vi "READBMSDYNDATA.vi"(8 "errin":errorcluster, 10 "set 400?":bool, 11 "Channel out":T1) -> (0 "errout":errorcluster, 3 "Data out":T2)   [LabVIEW 2020]
uses:
  PCAN Basic/Controls/Channel.ctl
  PCAN Basic/Controls/BaudrateEenum.ctl
  PCAN Basic/PCANBasic.lvlib
  Alex_Peak_lib/PEAK_lib_ALEX.lvlib
panel:
  out "F106 Power Distribution Status":string
  out "stop":bool
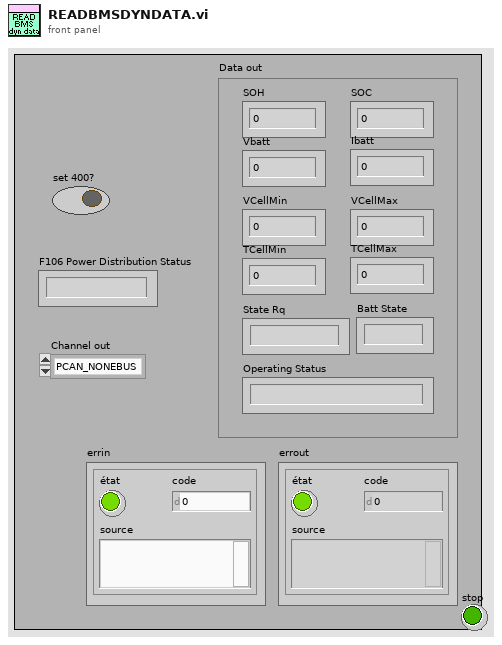
[diagram p1: front panel]
types:
  T1 = typedef "PCANBasic.lvlib/Channel.ctl" = enum16{"PCAN_NONEBUS", "not used1", "not used2", "not used3", "not used4", "not used5", "not used6", "not used7", "not used8", "not used9", "not used10", "not used11", "not used12", "not used13", "not used14", "not used15", "not used16", "not used17", "not used18", "not used19", "not used20", "not used21", "not used22", "not used23", "not used24", "not used25", "not used26", "not used27", "not used28", "not used29", "not used30", "not used31", "not used32", "PCAN_ISABUS1", "PCAN_ISABUS2", "PCAN_ISABUS3", "PCAN_ISABUS4", "PCAN_ISABUS5", "PCAN_ISABUS6", "PCAN_ISABUS7", "PCAN_ISABUS8", "not used41", "not used42", "not used43", "not used44", "not used45", "not used46", "not used47", "not used48", "PCAN_DNGBUS1", "not used50", "not used51", "not used52", "not used53", "not used54", "not used55", "not used56", "not used57", "not used58", "not used59", "not used60", "not used61", "not used62", "not used63", "not used64", "PCAN_PCIBUS1", "PCAN_PCIBUS2", "PCAN_PCIBUS3", "PCAN_PCIBUS4", "PCAN_PCIBUS5", "PCAN_PCIBUS6", "PCAN_PCIBUS7", "PCAN_PCIBUS8", "not used73", "not used74", "not used75", "not used76", "not used77", "not used78", "not used79", "not used80", "PCAN_USBBUS1", "PCAN_USBBUS2", "PCAN_USBBUS3", "PCAN_USBBUS4", "PCAN_USBBUS5", "PCAN_USBBUS6", "PCAN_USBBUS7", "PCAN_USBBUS8", "Not used89", "Not used90", "Not used91", "Not used92", "Not used93", "Not used94", "Not used95", "Not used96", "PCAN_PCCBUS1", "PCAN_PCCBUS2"}
  T2 = cluster{"SOH":dbl, "SOC":dbl, "Vbatt":u32, "Ibatt":dbl, "VCellMax":u32, "VCellMin":u32, "TCellMin":i32, "TCellMax":i32, "State Rq":string, "Batt State":string, "Operating Status":string}
  T3 = typedef "PCANBasic.lvlib/BaudrateEenum.ctl" = enum16{"CAN_Baud_1M", "CAN_Baud_800K", "CAN_BAUD_500K", "CAN_BAUD_250K", "CAN_BAUD_125K", "CAN_BAUD_100K", "CAN_BAUD_95K", "CAN_BAUD_83K", "CAN_BAUD_50K", "CAN_BAUD_47K", "CAN_BAUD_33K", "CAN_BAUD_20K", "CAN_BAUD_10K", "CAN_BAUD_5K", "User Baudrate"}
  T4 = cluster{"F400 Battery Charge Type":string, "F400 Battery State Request":string, "F400 Ext Insulation Test Control":string, "F400 Int Insulation Test Control":string, "F400 Vehicle Speed":i32, "F400 Ambiant Temperature":i32, "F400 Charger Available Power":i32, "F400 Count":i32, "F106 Keep Active request":string, "F106 Battery State":string, "F106 Operating Status":string, "F106 Battery SOC":dbl, "F106 Battery SOH":dbl, "F106 Ext Insulation Test Status":string, "F106 Int Insulation Test Status":string, "F106 Power Distribution Status":string, "F106 Power Switch Off Delay":i32, "F106 Power Switch Off Request":string, "F106 Count":i32, "F101 Battery Voltage":u32, "F101 Battery Current":dbl, "F101 Max Charge Current":u32, "F101 Max Discharge Current":u32, "F101 Max Discharge Current Temp Limit":string, "F101 Max Discharge Current SOC Limit":string, "F101 Max Charge Current Temp Limit":string, "F101 Max Charge Current SOC Limit":string, "F101 Deliverable Energy":dbl, "F101 Count":u32, "F102 Cell Average Voltage":u32, "F102 Cell Min Voltage":u32, "F102 Cell Max Voltage":u32, "F102 Cell Average Temp":i32, "F102 Cell Min Temp":i32, "F102 Count":u32, "F103 SumOfInternalResistanceT":i32, "F100 Charge Voltage Setpoint":i32, "F100 Charge Current Setpoint":dbl, "F100 Equilization Status":bool, "F100 Charge Competed":bool, "F100 Count":i32, "F107 Outlet Water Temp Request":i32, "F107 Outlet Water Temp Status":i32, "F107 Flow Rate Request":i32, "F107 Inlet Water Temp":i32, "F107 Ambiant Temperature 2":i32, "F105 Max Power Charge Continuous":i32, "F105 Max Power Charge Long Prediction":i32, "F105 Max Power Charge Short Prediction":i32, "F105 Max Current Charge Continuous":i32, "F105 Max Current Charge Short Prediction":i32, "F105 Count ":i32, "F104 Max Power Discharge Continuous":i32, "F104 Max Power Discharge Long Prediction":i32, "F104 Max Power Discharge Short Prediction":i32, "F104 Max Current Discharge Continuous":i32, "F104 Max Current Discharge Short Prediction":i32, "F104 Count ":i32, "F103 Count":i32, "F103 Cell Max Temp":i32, "F103 Max Current Discharge Long Prediction":i32, "F103 Max Current Charge Long Prediction":i32, "F107 Count":i32}
  T5 = cluster{"ID":u32, "MSGTYPE":u8, "LEN":u8, "DATA[0]":u8, "DATA[1]":u8, "DATA[2]":u8, "DATA[3]":u8, "DATA[4]":u8, "DATA[5]":u8, "DATA[6]":u8, "DATA[7]":u8}
  T6 = cluster{"F400 Battery Charge Type":string, "F400 Battery State Request":string, "F400 Ext Insulation Test Control":string, "F400 Int Insulation Test Control":string, "F400 Vehicle Speed":i32, "F400 Ambiant Temperature":i32, "F400 Charger Available Power":i32, "F400 Count":i32, "F106 Keep Active request":string, "F106 Battery State":string, "F106 Operating Status":string, "F106 Battery SOC":dbl, "F106 Battery SOH":dbl, "F106 Ext Insulation Test Status":string, "F106 Int Insulation Test Status":string, "F106 Power Distribution Status":string, "F106 Power Switch Off Delay":i32, "F106 Power Switch Off Request":string, "F106 Count":i32, "F101 Battery Voltage":u32, "F101 Battery Current":dbl, "F101 Max Charge Current":u32, "F101 Max Discharge Current":u32, "F101 Max Discharge Current Temp Limit":string, "F101 Max Discharge Current SOC Limit":string, "F101 Max Charge Current Temp Limit":string, "F101 Max Charge Current SOC Limit":string, "F101 Deliverable Energy":dbl, "F101 Count":u32, "F102 Cell Average Voltage":u32, "F102 Cell Min Voltage":u32, "F102 Cell Max Voltage":u32, "F102 Cell Average Temp":i32, "F102 Cell Min Temp":i32, "F102 Count":u32, "F103 SumOfInternalResistanceT":i32, "F100 Charge Voltage Setpoint":i32, "F100 Charge Current Setpoint":i32, "F100 Equilization Status":bool, "F100 Charge Competed":bool, "F100 Count":i32, "F107 Outlet Water Temp Request":i32, "F107 Outlet Water Temp Status":i32, "F107 Flow Rate Request":i32, "F107 Inlet Water Temp":i32, "F107 Ambiant Temperature 2":i32, "F105 Max Power Charge Continuous":i32, "F105 Max Power Charge Long Prediction":i32, "F105 Max Power Charge Short Prediction":i32, "F105 Max Current Charge Continuous":i32, "F105 Max Current Charge Short Prediction":i32, "F105 Count ":i32, "F104 Max Power Discharge Continuous":i32, "F104 Max Power Discharge Long Prediction":i32, "F104 Max Power Discharge Short Prediction":i32, "F104 Max Current Discharge Continuous":i32, "F104 Max Current Discharge Short Prediction":i32, "F104 Count ":i32, "F103 Count":i32, "F103 Cell Max Temp":i32, "F103 Max Current Discharge Long Prediction":i32, "F103 Max Current Charge Long Prediction":i32, "F107 Count":i32}
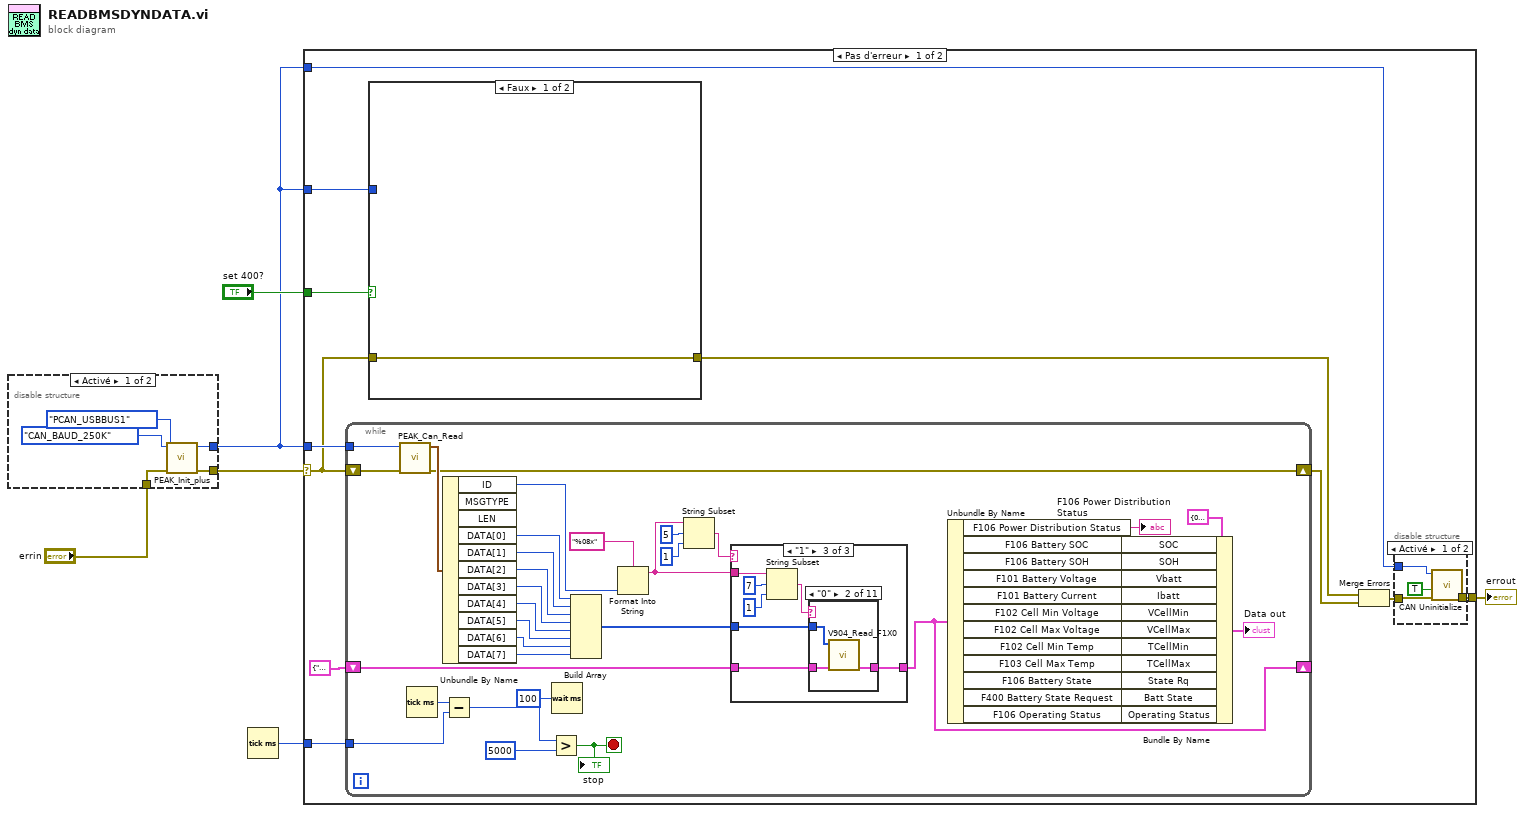
[diagram p0: block diagram]
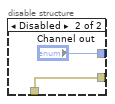
[diagram p2: hidden frame]
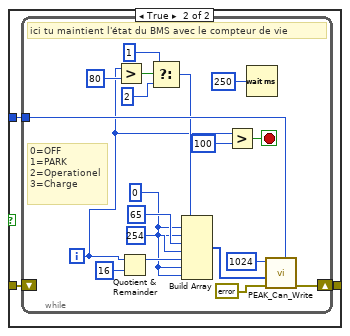
[diagram p4: hidden frame]
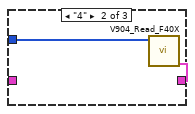
[diagram p6: hidden frame]
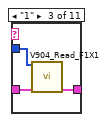
[diagram p8: hidden frame]
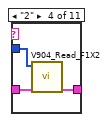
[diagram p9: hidden frame]
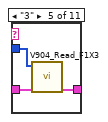
[diagram p10: hidden frame]
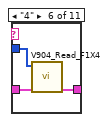
[diagram p11: hidden frame]
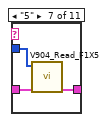
[diagram p12: hidden frame]
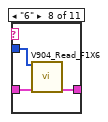
[diagram p13: hidden frame]
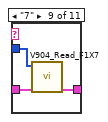
[diagram p14: hidden frame]
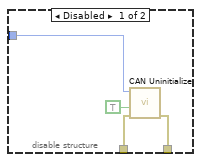
[diagram p18: hidden frame]
diagram:
  n1 = disable-structure shown="Activé" {
    disable-tunnel: [w10 w12] -> w6
    disable-tunnel: "errin" -> [w9 w12]
    disable-tunnel: [w8 "Channel out"] -> w1
    frame Enabled {
      n2 = call "PEAK_Init_plus.vi"("errin"=w9, "Channel"=Channel."PCAN_USBBUS1", "BTR0BTR1"=BaudrateEenum."CAN_BAUD_250K") -> ("errout"=w10:errorcluster, "Channel out"=w8:T1)  [unwired: 7 in]
    }
    frame Disabled {
    }
  }
  n3 = Tick Count (ms)() -> (millisecond timer value=w3:u32)
  n4 = case shown="Pas d'erreur" w6 {
    selector: w6 -> [w20 w133]
    tunnel: w1 -> [w24 w131]
    tunnel: [w21 w132] -> w5
    tunnel: w3 -> [w22 _]
    tunnel: "set 400?" -> [w19 _]
    tunnel: w1 -> [w15 _]
    tunnel: w1 -> [w14 _]
    frame No Error {
      n5 = while {
        tunnel: w24 -> [w55]
        shift-right: [w61] -> _
        shift-left: T4 {"F400 Battery Charge Type"="", "F400 Battery State Request"="", "F400 Ext Insulation Test Control"="", "F400 Int Insulation Test Control"="", "F400 Vehicle Speed"=0, "F400 Ambiant Temperature"=0, "F400 Charger Available Power"=0, "F400 Count"=0, "F106 Keep Active request"="", "F106 Battery State"="", "F106 Operating Status"="", "F106 Battery SOC"=0.0, "F106 Battery SOH"=0.0, "F106 Ext Insulation Test Status"="", "F106 Int Insulation Test Status"="", "F106 Power Distribution Status"="", "F106 Power Switch Off Delay"=0, "F106 Power Switch Off Request"="", "F106 Count"=0, "F101 Battery Voltage"=0, "F101 Battery Current"=0.0, "F101 Max Charge Current"=0, "F101 Max Discharge Current"=0, "F101 Max Discharge Current Temp Limit"="", "F101 Max Discharge Current SOC Limit"="", "F101 Max Charge Current Temp Limit"="", "F101 Max Charge Current SOC Limit"="", "F101 Deliverable Energy"=0.0, "F101 Count"=0, "F102 Cell Average Voltage"=0, "F102 Cell Min Voltage"=0, "F102 Cell Max Voltage"=0, "F102 Cell Average Temp"=0, "F102 Cell Min Temp"=0, "F102 Count"=0, "F103 SumOfInternalResistanceT"=0, "F100 Charge Voltage Setpoint"=0, "F100 Charge Current Setpoint"=0.0, "F100 Equilization Status"=FALSE, "F100 Charge Competed"=FALSE, "F100 Count"=0, "F107 Outlet Water Temp Request"=0, "F107 Outlet Water Temp Status"=0, "F107 Flow Rate Request"=0, "F107 Inlet Water Temp"=0, "F107 Ambiant Temperature 2"=0, "F105 Max Power Charge Continuous"=0, "F105 Max Power Charge Long Prediction"=0, "F105 Max Power Charge Short Prediction"=0, "F105 Max Current Charge Continuous"=0, "F105 Max Current Charge Short Prediction"=0, "F105 Count "=0, "F104 Max Power Discharge Continuous"=0, "F104 Max Power Discharge Long Prediction"=0, "F104 Max Power Discharge Short Prediction"=0, "F104 Max Current Discharge Continuous"=0, "F104 Max Current Discharge Short Prediction"=0, "F104 Count "=0, "F103 Count"=0, "F103 Cell Max Temp"=0, "F103 Max Current Discharge Long Prediction"=0, "F103 Max Current Charge Long Prediction"=0, "F107 Count"=0} ("cluster de sortie") -> [w77]
        shift-right: [w75] -> w16
        shift-left: w20 -> [w54]
        tunnel: w22 -> [w59]
        stop <- w56 stop-if-true
        n6 = call "PEAK_Can_Read.vi"("errin"=w54, "Channel out"=w55) -> ("errout"=w75:errorcluster, "MessageBuffer out"=w93:T5)  [unwired: 7 in, 1 out]
        n7 = Tick Count (ms)() -> (millisecond timer value=w60:u32)
        n8 = Unbundle By Name(w93) -> ("ID"=w87:u32, "DATA[0]"=w86:u8, "DATA[1]"=w85:u8, "DATA[2]"=w84:u8, "DATA[3]"=w83:u8, "DATA[4]"=w82:u8, "DATA[5]"=w81:u8, "DATA[6]"=w80:u8, "DATA[7]"=w79:u8)  [unwired: 2 out]
        n9 = Subtract(x=w60, y=w59) -> (x-y=w58:u32)
        n10 = Greater?(x=w58, y=u32 5000) -> (0:w56:bool)
        "stop" <- w56
        n11 = Wait (ms)(milliseconds to wait=u32 100 ("attente (ms)")) -> ()  [unwired: 1 out]
        n12 = Build Array(w86, w85, w84, w83, w82, w81, w80, w79) -> (w78:u8[])
        n13 = Format Into String(format string="%08x", w87) -> (resulting string=w91:string)  [unwired: 2 in, 1 out]
        n14 = String Subset(string=w91, offset (0)=5, length (rest)=1 ("longueur (reste)")) -> (substring=w90:string)
        n15 = case shown="\"1\"" w90 {
          tunnel: w77 -> [w94 _ w98]
          tunnel: w78 -> [_ w96 w103]
          tunnel: [w94 w95 w97] -> w61
          tunnel: w91 -> [_ _ w99]
          frame "Faux", Default {
          }
          frame "4" {
            n16 = call "V904_Read_F40X.vi"("Data"=w96) -> ("cluster de sortie"=w95:T4)  [unwired: 10 in]
          }
          frame "1" {
            n17 = String Subset(string=w99, offset (0)=7, length (rest)=1 ("longueur (reste)")) -> (substring=w100:string)
            n18 = case shown="\"0\"" w100 {
              tunnel: w103 -> [_ w107 w109 w113 w116 w119 w122 w125 w128 _ _]
              tunnel: w98 -> [w104 w106 w110 w112 w115 w118 w121 w124 w127 w129 w130]
              tunnel: [w104 w105 w108 w111 w114 w117 w120 w123 w126 w129 w130] -> w97
              frame "Faux", Default {
              }
              frame "0" {
                n19 = call "V904_Read_F1X0.vi"("cluster input"=w106, "Data"=w107) -> ("cluster de sortie"=w105:T6)  [unwired: 9 in]
              }
              frame "1" {
                n20 = call "V904_Read_F1X1.vi"("Data"=w109, "cluster input"=w110) -> ("cluster de sortie"=w108:T4)  [unwired: 13 in]
              }
              frame "2" {
                n21 = call "V904_Read_F1X2.vi"("cluster input"=w112, "Data"=w113) -> ("cluster de sortie"=w111:T4)  [unwired: 9 in]
              }
              frame "3" {
                n22 = call "V904_Read_F1X3.vi"("cluster input"=w115, "Data"=w116) -> ("cluster de sortie"=w114:T4)  [unwired: 9 in]
              }
              frame "4" {
                n23 = call "V904_Read_F1X4.vi"("cluster input"=w118, "Data"=w119) -> ("cluster de sortie"=w117:T4)  [unwired: 9 in]
              }
              frame "5" {
                n24 = call "V904_Read_F1X5.vi"("cluster input"=w121, "Data"=w122) -> ("cluster de sortie"=w120:T4)  [unwired: 9 in]
              }
              frame "6" {
                n25 = call "V904_Read_F1X6.vi"("Data"=w125, "cluster input"=w124) -> ("cluster de sortie"=w123:T4)  [unwired: 13 in]
              }
              frame "7" {
                n26 = call "V904_Read_F1X7.vi"("cluster input"=w127, "Data"=w128) -> ("cluster de sortie"=w126:T4)  [unwired: 9 in]
              }
              frame "8" {
              }
              frame "9" {
              }
            }
          }
        }
        n27 = Unbundle By Name(w61) -> ("F106 Power Distribution Status"=→"F106 Power Distribution Status":string, "F106 Battery SOC"=w73:dbl, "F106 Battery SOH"=w72:dbl, "F101 Battery Voltage"=w71:u32, "F101 Battery Current"=w70:dbl, "F102 Cell Min Voltage"=w69:u32, "F102 Cell Max Voltage"=w68:u32, "F102 Cell Min Temp"=w67:i32, "F103 Cell Max Temp"=w66:i32, "F106 Battery State"=w65:string, "F400 Battery State Request"=w64:string, "F106 Operating Status"=w63:string)
        n28 = Bundle By Name(cluster=T2 {"SOH"=0.0, "SOC"=0.0, "Vbatt"=0, "Ibatt"=0.0, "VCellMax"=0, "VCellMin"=0, "TCellMin"=0, "TCellMax"=0, "State Rq"="", "Batt State"="", "Operating Status"=""} ("Data out"), "SOC"=w73, "SOH"=w72, "Vbatt"=w71, "Ibatt"=w70, "VCellMin"=w69, "VCellMax"=w68, "TCellMin"=w67, "TCellMax"=w66, "State Rq"=w65, "Batt State"=w64, "Operating Status"=w63) -> (→"Data out":T2)
      }
      n29 = case shown="Faux" w19 {
        tunnel: w20 -> [w30 w33]
        tunnel: [w30 w32] -> w17
        tunnel: w15 -> [_ w31]
        frame False {
        }
        frame True {
          n30 = while {
            shift-right: [w52] -> w32
            shift-left: w33 -> [_]
            tunnel: w31 -> [w42]
            i -> [w36]
            stop <- w34 stop-if-true
            w43 = u8 0
            # "0=OFF\n1=PARK\n2=Operationel\n3=Charge"
            # "ici tu maintient l'état du BMS avec le compteur de vie"
            n31 = Greater?(x=w36, y=80) -> (0:w40:bool)
            n32 = Quotient & Remainder(x=w36, y=16) -> (x-y*floor(x/y)=w45:i32)  [unwired: 1 out]
            n33 = Select(t=1 ("cas vrai"), s=w40, f=2 ("élément")) -> (s? t:f=w37:i32)
            n34 = Build Array(w37, w43, w43, u8 65, u8 254, w45, w43, w43) -> (w46:i32[])
            n35 = Greater?(x=w36, y=100) -> (0:w34:bool)
            n36 = Wait (ms)(milliseconds to wait=u32 250 ("attente (ms)")) -> ()  [unwired: 1 out]
            n37 = call "PEAK_Can_Write.vi"("CAN Handle"=w42, "errin"=errorcluster {"status"=FALSE, "code"=0, "source"=""} ("errout"), "CAN Data"=w46, "Identifier"=u32 1024) -> ("errout"=w52:errorcluster)  [unwired: 7 in]
          }
        }
      }
      n38 = Merge Errors(w17, w16) -> (w18:errorcluster)
      n39 = disable-structure shown="Activé" {
        disable-tunnel: [w27 w29] -> w21
        disable-tunnel: w18 -> [w26 w29]
        disable-tunnel: w14 -> [w25 _]
        frame Enabled {
          n40 = call "CAN Uninitialize.vi"("error in (no error)"=w26, "Ignore input error"=TRUE, "Channel"=w25) -> ("error out"=w27:errorcluster)  [unwired: 6 in, 2 out]
        }
        frame Disabled {
        }
      }
    }
    frame Error {
      n41 = disable-structure shown="Activé" {
        disable-tunnel: w133 -> [w137 w138]
        disable-tunnel: [w136 w138] -> w132
        disable-tunnel: w131 -> [w134 _]
        frame Disabled {
          n42 = call "CAN Uninitialize.vi"("error in (no error)"=w137, "Ignore input error"=TRUE, "Channel"=w134) -> ("error out"=w136:errorcluster)  [unwired: 6 in, 2 out]
        }
        frame Enabled {
        }
      }
    }
  }
  "errout" <- w5
